vi "Streamline1005.vi"   [LabVIEW 2013]
uses:
  <vilib>/Heliosphere Research LLC/Advanced Plotting Toolkit/api_plotting/StreamlineProperties.ctl
  <vilib>/Heliosphere Research LLC/Advanced Plotting Toolkit/properties/Line.ctl
  <vilib>/Heliosphere Research LLC/Advanced Plotting Toolkit/properties/Line_Style.ctl
  <vilib>/Heliosphere Research LLC/Advanced Plotting Toolkit/typedefs/PlotColor.ctl
  <vilib>/Heliosphere Research LLC/Advanced Plotting Toolkit/properties/Colormap.ctl
  <vilib>/Heliosphere Research LLC/Advanced Plotting Toolkit/properties/Colormap_Map.ctl
  <vilib>/Heliosphere Research LLC/Advanced Plotting Toolkit/properties/Colormap_Scaling.ctl
  <vilib>/Heliosphere Research LLC/Advanced Plotting Toolkit/Advanced Plotting Toolkit.lvlib
types:
  T1 = typedef "Advanced Plotting Toolkit.lvlib/Line_Style.ctl" = enum16{"Automatic", "Solid", "Dashed", "Dotted", "Dash-dot", "Invisible"}
  T2 = typedef "Advanced Plotting Toolkit.lvlib/StreamlineProperties.ctl" = cluster{"Density":dbl, "Arrow Size":dbl, "Line":T3, "Colormap":T5}
  T3 = typedef "Advanced Plotting Toolkit.lvlib/Line.ctl" = cluster{"Style":T1, "Color":T4, "Width":sgl}
  T4 = typedef "Advanced Plotting Toolkit.lvlib/PlotColor.ctl" = u32
  T5 = typedef "Advanced Plotting Toolkit.lvlib/Colormap.ctl" = cluster{"Map":T6, "Value Min":dbl, "Value Max":dbl, "Scaling":T7, "Reverse":bool}
  T6 = typedef "Advanced Plotting Toolkit.lvlib/Colormap_Map.ctl" = enum16{"Automatic", "Rainbow", "Hot and Cold", "White-Black", "White-Blue", "White-Green", "White-Red", "Fire", "Water", "Earth", "Air", "Pastel", "Banded", "Stepped"}
  T7 = typedef "Advanced Plotting Toolkit.lvlib/Colormap_Scaling.ctl" = enum16{"Default"}
  T8 = typedef "Advanced Plotting Toolkit.lvlib/PlotID.ctl" = i32
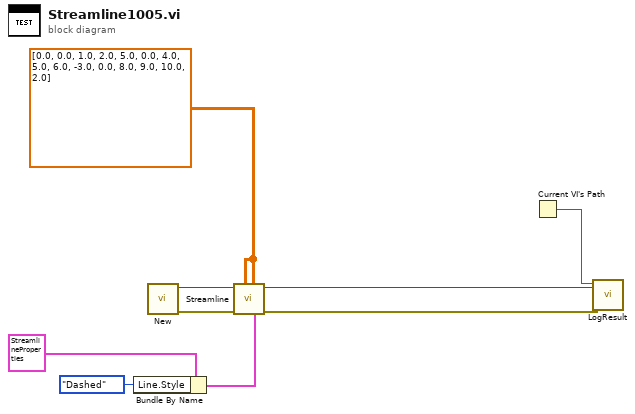
[diagram p0: block diagram]
diagram:
  w2 = dbl[][] [[0.0, 0.0, 1.0, 2.0, 5.0], [0.0, 4.0, 5.0, 6.0, -3.0], [0.0, 8.0, 9.0, 10.0, 2.0]] ("Data")
  n1 = Bundle By Name(cluster=T2 {"Density"=nan, "Arrow Size"=nan, "Line"={"Style"=enum."Automatic", "Color"=2147483647, "Width"=nan}, "Colormap"={"Map"=enum."Automatic", "Value Min"=nan, "Value Max"=nan, "Scaling"=enum."Default", "Reverse"=FALSE}} ("Streamline Properties"), "Line.Style"=Line_Style."Dashed") -> (w3:T2)
  n2 = call <vilib>:"New.vi"() -> ("error out"=w7:errorcluster, "Plot ID"=w8:T8)  [unwired: 10 in]
  n3 = call <vilib>:"Streamline.vi"("Properties"=w3, "Y Vector Component"=w2, "X Vector Component"=w2, "error in (no error)"=w7, "Plot ID"=w8) -> ("error out"=w5:errorcluster, "Plot ID Out"=w6:T8)  [unwired: 5 in]
  n4 = Current VI's Path() -> (path=w9:path)
  n5 = call "LogResult.vi"("Test Result"=w5, "Test Artifact"=w6, "VI Path"=w9) -> ()  [unwired: 9 in]
